vi "Run.vi"(8 "error in (no error)":errorcluster, 9 "Penalty":dbl, 10 "Maze":i32[][](array[numeric]), 11 "Runner in":refnum<class "Sentinel.lvclass">) -> (0 "error out":errorcluster, 1 "Direction":T1, 2 "Action":T2, 3 "Runner out":refnum<class "Sentinel.lvclass">, 4 "Replicated":refnum<class "Square.lvclass">)   [LabVIEW 2015, in "Sentinel.lvclass"]
uses:
  Sentinel.lvclass
  Type Defs/Action Enum.ctl
  Type Defs/Direction Enum.ctl
  Square/Square.lvclass
  Carl/Formics/Attack Options.ctl
  Sentinel.lvclass/Sentinel.ctl
  SubVIs/Read-Only Globals.vi
  Type Defs/SB Type Defs.lvlib
  Carl/Common/Common.lvlib
  Carl/Formics/Formics.lvclass
panel:
  # "NOTICE - YOU MUST NOT REMOVE THIS NOTICE. PER THE FOLLOWING LICENSE, YOU MAY REPRODUCE THIS SOFTWARE PROVIDED YOU FOLLOW THE TERMS\nOF THE LICENSE.\n\n---BEGIN BSD LICENSE (http://opensource.org/licenses/BSD-2-Clause)---\nCopyright (c) 2015, Endigit, Inc. <robert@endigit.com>\nAll rights reserved.\n\nRedistribution and use in source and binary forms, with or without modification, are permitted provided that the following conditions are met:\n\n1. Redistributions of source code must retain the above copyright notice, this list of conditions and the following disclaimer.\n\n2. Redistributions in binary form must reproduce the above copyright notice, this list of conditions and the following disclaimer in the documentation and/or other \nmaterials provided with the distribution.\n\nTHIS SOFTWARE IS PROVIDED BY THE COPYRIGHT HOLDERS AND CONTRIBUTORS \"AS IS\" AND ANY EXPRESS OR IMPLIED WARRANTIES, INCLUDING, BUT NOT \nLIMITED TO, THE IMPLIED WARRANTIES OF MERCHANTABILITY AND FITNESS FOR A PARTICULAR PURPOSE ARE DISCLAIMED. IN NO EVENT SHALL THE COPYRIGHT \nHOLDER OR CONTRIBUTORS BE LIABLE FOR ANY DIRECT, INDIRECT, INCIDENTAL, SPECIAL, EXEMPLARY, OR CONSEQUENTIAL DAMAGES (INCLUDING, BUT NOT \nLIMITED TO, PROCUREMENT OF SUBSTITUTE GOODS OR SERVICES; LOSS OF USE, DATA, OR PROFITS; OR BUSINESS INTERRUPTION) HOWEVER CAUSED AND ON \nANY THEORY OF LIABILITY, WHETHER IN CONTRACT, STRICT LIABILITY, OR TORT (INCLUDING NEGLIGENCE OR OTHERWISE) ARISING IN ANY WAY OUT OF THE USE \nOF THIS SOFTWARE, EVEN IF ADVISED OF THE POSSIBILITY OF SUCH DAMAGE.\n---END BSD LICENSE---"
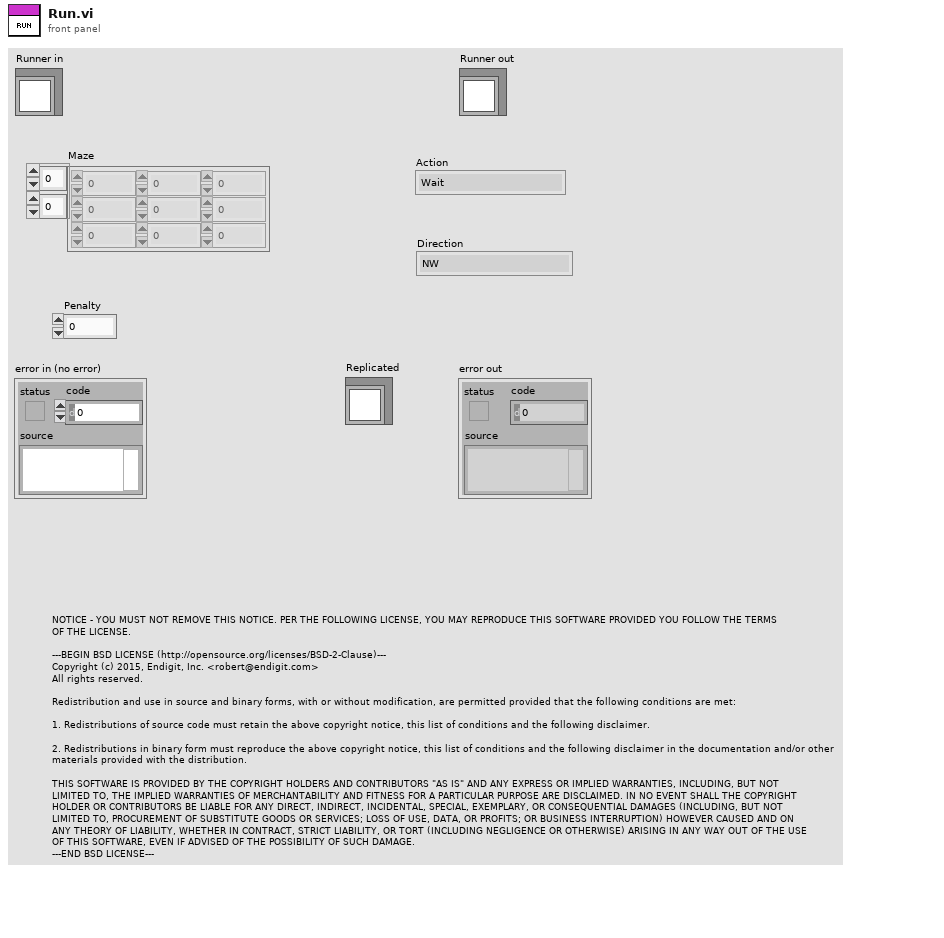
[diagram p1: front panel]
types:
  T1 = typedef "SB Type Defs.lvlib/Direction Enum.ctl" = enum16{"NW", "N", "NE", "E", "SE", "S", "SW", "W"}
  T2 = typedef "SB Type Defs.lvlib/Action Enum.ctl" = enum16{"Wait", "Move", "Attack", "Replicate"}
  T3 = typedef "Formics.lvclass/Attack Options.ctl" = enum16{"Attack", "Run", "Distract"}
  T4 = enum16{"Replicator", "Replicatee", "Eastwards", "Westwards"}
  T5 = enum16{"Replication", "Northwards", "Southwards"}
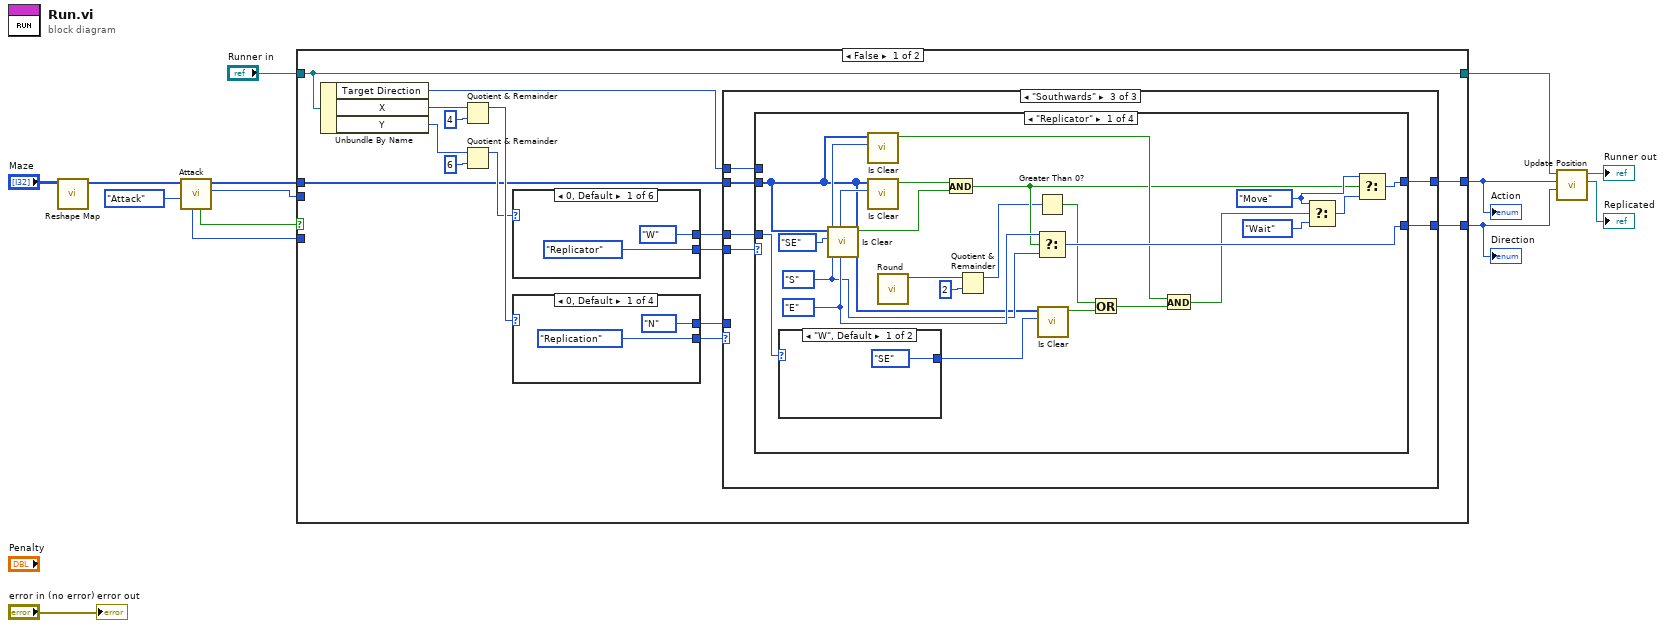
[diagram p0: block diagram]
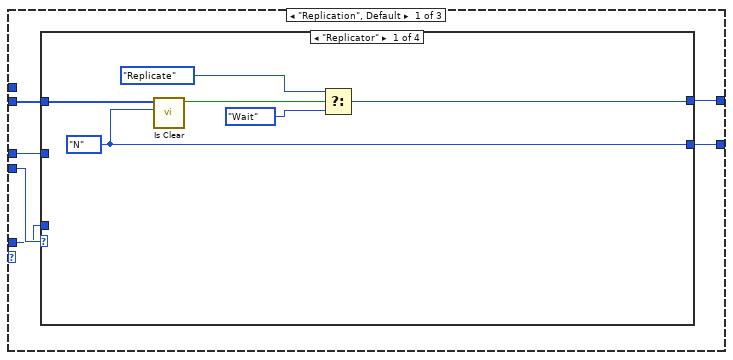
[diagram p2: hidden frame]
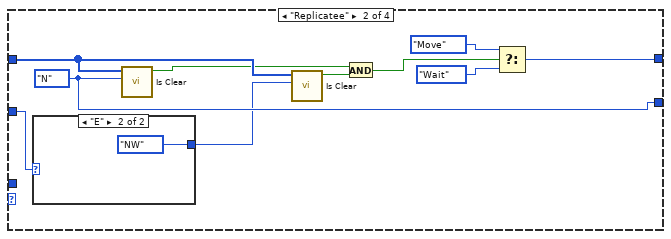
[diagram p3: hidden frame]
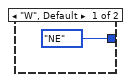
[diagram p4: hidden frame]
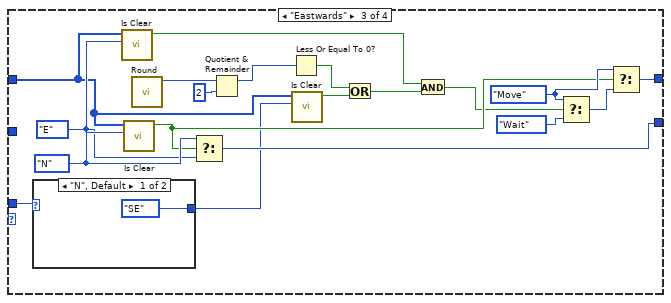
[diagram p5: hidden frame]
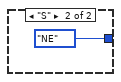
[diagram p6: hidden frame]
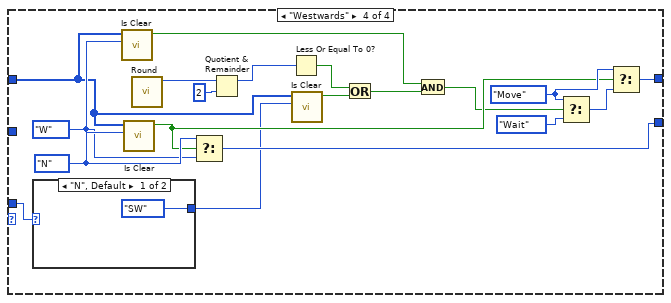
[diagram p7: hidden frame]
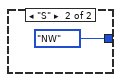
[diagram p8: hidden frame]
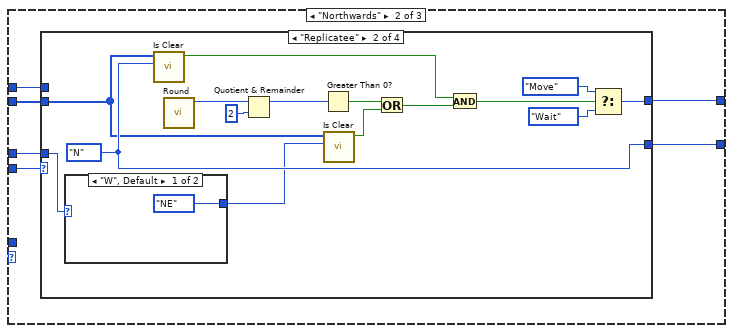
[diagram p9: hidden frame]
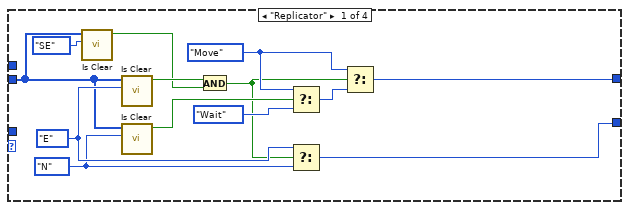
[diagram p10: hidden frame]
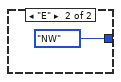
[diagram p11: hidden frame]
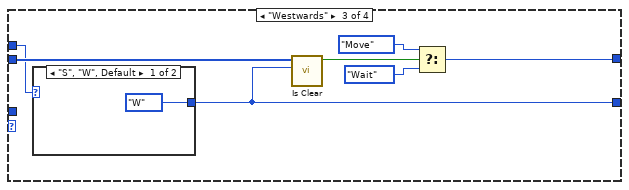
[diagram p12: hidden frame]
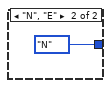
[diagram p13: hidden frame]
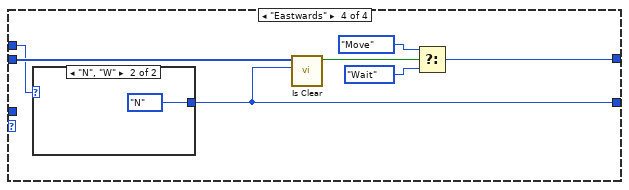
[diagram p14: hidden frame]
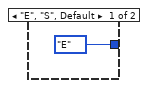
[diagram p15: hidden frame]
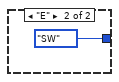
[diagram p16: hidden frame]
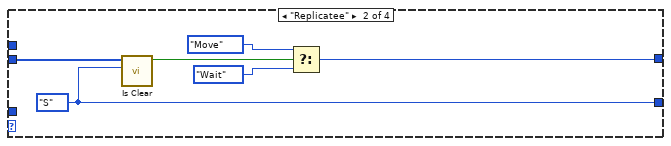
[diagram p17: hidden frame]
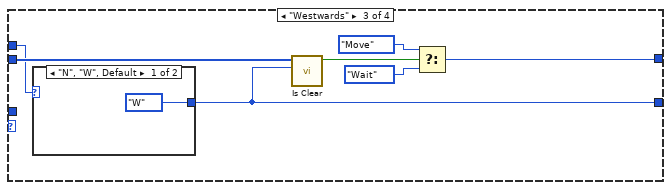
[diagram p18: hidden frame]
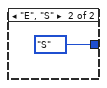
[diagram p19: hidden frame]
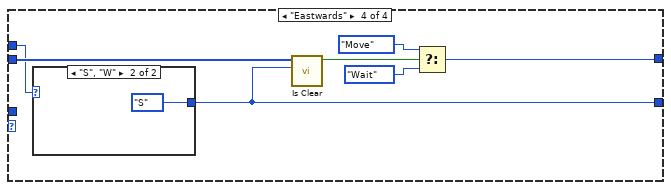
[diagram p20: hidden frame]
diagram:
  n1 = call "Reshape Map.vi"("Maze (0: Empty, -1: Enemy. >0: Teammate"="Maze") -> ("Map"=w12:i32[])  [unwired: 9 in, 1 out]
  n2 = call "Attack.vi"("Attack?"=Attack_Options."Attack", "Maze (0: Empty, -1: Enemy. >0: Teammate"=w12) -> ("Action"=w10:T2, "Maze (0: Empty, -1: Enemy. >0: Teammate 2"=w7:i32[], "Enemy Found?"=w11:bool, "Enemy Direction"=w9:i32)  [unwired: 4 in, 2 out]
  n3 = case shown="False" w11 {
    tunnel: "Runner in" -> [w21 w224]
    tunnel: w10 -> [_ w226]
    tunnel: [w20 w226] -> w1
    tunnel: w9 -> [_ w225]
    tunnel: [w19 w225] -> w2
    tunnel: [w21 w224] -> w5
    tunnel: w7 -> [w18 _]
    frame False {
      n4 = Unbundle By Name(w21) -> ("Target Direction"=w16:T1, "X"=w29:i16, "Y"=w25:i16)
      n5 = Quotient & Remainder(x=w29, y=4) -> (x-y*floor(x/y)=w27:i32)  [unwired: 1 out]
      n6 = Quotient & Remainder(x=w25, y=6) -> (x-y*floor(x/y)=w24:i32)  [unwired: 1 out]
      n7 = case shown="0, Default" w24 {
        tunnel: [T4."Replicator" ("Rows") T4."Replicatee" ("Rows") T4."Eastwards" ("Rows") T4."Replicator" ("Rows") T4."Replicatee" ("Rows") T4."Westwards" ("Rows")] -> w22
        tunnel: [Direction_Enum."W" ("Direction") Direction_Enum."E" ("Direction") Direction_Enum."E" ("Direction") Direction_Enum."E" ("Direction") Direction_Enum."W" ("Direction") Direction_Enum."W" ("Direction")] -> w17
        frame 0, Default {
        }
        frame 1 {
        }
        frame 2 {
        }
        frame 3 {
        }
        frame 4 {
        }
        frame 5 {
        }
      }
      n8 = case shown="0, Default" w27 {
        tunnel: [Direction_Enum."N" ("Direction") Direction_Enum."N" ("Direction") Direction_Enum."S" ("Direction") Direction_Enum."S" ("Direction")] -> w15
        tunnel: [T5."Replication" ("Cols") T5."Northwards" ("Cols") T5."Replication" ("Cols") T5."Southwards" ("Cols")] -> w23
        frame 0, Default {
        }
        frame 1 {
        }
        frame 2 {
        }
        frame 3 {
        }
      }
      n9 = case shown="\"Southwards\"" w23 {
        tunnel: w22 -> [w35 w101 w155]
        tunnel: [w34 w100 w154] -> w20
        tunnel: [w33 w99 w153] -> w19
        tunnel: w18 -> [w32 w98 w152]
        tunnel: w17 -> [w31 w97 w151]
        tunnel: w16 -> [_ w96 w150]
        tunnel: w15 -> [w30 _ _]
        frame "Replication", Default {
          n10 = case shown="\"Replicator\"" w35 {
            tunnel: [w38 w48 w72 w93] -> w34
            tunnel: [w40 w51 w69 w90] -> w33
            tunnel: w32 -> [w41 w46 w55 w80]
            tunnel: w31 -> [_ w47 _ _]
            tunnel: w30 -> [_ _ w54 w75]
            frame "Replicator" {
              w40 = Direction_Enum."N" ("Direction")
              n11 = call "Is Clear.vi"("Direction"=w40, "Maze (0: Empty, -1: Enemy. >0: Teammate in"=w41) -> ("Is Clear"=w36:bool)  [unwired: 9 in]
              n12 = Select(t=Action_Enum."Replicate" ("Action"), s=w36, f=Action_Enum."Wait" ("Action")) -> (s? t:f=w38:T2)
            }
            frame "Replicatee" {
              w51 = Direction_Enum."N" ("Direction")
              n13 = case shown="\"E\"" w47 {
                tunnel: [Direction_Enum."NE" ("Direction") Direction_Enum."NW" ("Direction")] -> w45
                frame "W", Default {
                }
                frame "E" {
                }
              }
              n14 = call "Is Clear.vi"("Direction"=w51, "Maze (0: Empty, -1: Enemy. >0: Teammate in"=w46) -> ("Is Clear"=w43:bool)  [unwired: 9 in]
              n15 = call "Is Clear.vi"("Direction"=w45, "Maze (0: Empty, -1: Enemy. >0: Teammate in"=w46) -> ("Is Clear"=w44:bool)  [unwired: 9 in]
              n16 = And(x=w43, y=w44) -> (x .and. y?=w42:bool)
              n17 = Select(t=Action_Enum."Move" ("Action"), s=w42, f=Action_Enum."Wait" ("Action")) -> (s? t:f=w48:T2)
            }
            frame "Eastwards" {
              w70 = Direction_Enum."E" ("Direction")
              w67 = Action_Enum."Move" ("Action")
              w71 = Direction_Enum."N" ("Direction")
              n18 = case shown="\"N\", Default" w54 {
                tunnel: [Direction_Enum."SE" ("Direction") Direction_Enum."NE" ("Direction")] -> w60
                frame "N", Default {
                }
                frame "S" {
                }
              }
              n19 = call "Is Clear.vi"("Direction"=w70, "Maze (0: Empty, -1: Enemy. >0: Teammate in"=w55) -> ("Is Clear"=w59:bool)  [unwired: 9 in]
              n20 = call "Is Clear.vi"("Direction"=w71, "Maze (0: Empty, -1: Enemy. >0: Teammate in"=w55) -> ("Is Clear"=w65:bool)  [unwired: 9 in]
              n21 = call "Round.vi"() -> ("Round"=w64:i32)  [unwired: 11 in]
              n22 = Select(t=w71, s=w65, f=w70) -> (s? t:f=w69:T1)
              n23 = Quotient & Remainder(x=w64, y=2) -> (x-y*floor(x/y)=w62:i32)  [unwired: 1 out]
              n24 = Less Or Equal To 0?(x=w62) -> (x <= 0?=w61:bool)
              n25 = call "Is Clear.vi"("Direction"=w60, "Maze (0: Empty, -1: Enemy. >0: Teammate in"=w55) -> ("Is Clear"=w58:bool)  [unwired: 9 in]
              n26 = Or(x=w61, y=w58) -> (x .or. y?=w57:bool)
              n27 = And(x=w59, y=w57) -> (x .and. y?=w56:bool)
              n28 = Select(t=w67, s=w56, f=Action_Enum."Wait" ("Action")) -> (s? t:f=w66:T2)
              n29 = Select(t=w67, s=w65, f=w66) -> (s? t:f=w72:T2)
            }
            frame "Westwards" {
              w91 = Direction_Enum."W" ("Direction")
              w88 = Action_Enum."Move" ("Action")
              w92 = Direction_Enum."N" ("Direction")
              n30 = case shown="\"N\", Default" w75 {
                tunnel: [Direction_Enum."SW" ("Direction") Direction_Enum."NW" ("Direction")] -> w81
                frame "N", Default {
                }
                frame "S" {
                }
              }
              n31 = call "Is Clear.vi"("Direction"=w91, "Maze (0: Empty, -1: Enemy. >0: Teammate in"=w80) -> ("Is Clear"=w79:bool)  [unwired: 9 in]
              n32 = call "Is Clear.vi"("Direction"=w92, "Maze (0: Empty, -1: Enemy. >0: Teammate in"=w80) -> ("Is Clear"=w86:bool)  [unwired: 9 in]
              n33 = call "Round.vi"() -> ("Round"=w84:i32)  [unwired: 11 in]
              n34 = Select(t=w92, s=w86, f=w91) -> (s? t:f=w90:T1)
              n35 = Quotient & Remainder(x=w84, y=2) -> (x-y*floor(x/y)=w83:i32)  [unwired: 1 out]
              n36 = Less Or Equal To 0?(x=w83) -> (x <= 0?=w82:bool)
              n37 = call "Is Clear.vi"("Direction"=w81, "Maze (0: Empty, -1: Enemy. >0: Teammate in"=w80) -> ("Is Clear"=w78:bool)  [unwired: 9 in]
              n38 = Or(x=w82, y=w78) -> (x .or. y?=w77:bool)
              n39 = And(x=w79, y=w77) -> (x .and. y?=w76:bool)
              n40 = Select(t=w88, s=w76, f=Action_Enum."Wait" ("Action")) -> (s? t:f=w87:T2)
              n41 = Select(t=w88, s=w86, f=w87) -> (s? t:f=w93:T2)
            }
          }
        }
        frame "Northwards" {
          n42 = case shown="\"Replicatee\"" w101 {
            tunnel: [w109 w126 w135 w144] -> w100
            tunnel: [w110 w127 w132 w141] -> w99
            tunnel: w98 -> [w108 w125 w134 w143]
            tunnel: w97 -> [_ w123 _ _]
            tunnel: w96 -> [_ _ w133 w142]
            frame "Replicator" {
              w103 = Direction_Enum."N" ("Direction")
              w111 = Direction_Enum."E" ("Direction")
              w106 = Action_Enum."Move" ("Action")
              n43 = call "Is Clear.vi"("Direction"=Direction_Enum."SE", "Maze (0: Empty, -1: Enemy. >0: Teammate in"=w108) -> ("Is Clear"=w112:bool)  [unwired: 9 in]
              n44 = call "Is Clear.vi"("Direction"=w111, "Maze (0: Empty, -1: Enemy. >0: Teammate in"=w108) -> ("Is Clear"=w113:bool)  [unwired: 9 in]
              n45 = call "Is Clear.vi"("Direction"=w103, "Maze (0: Empty, -1: Enemy. >0: Teammate in"=w108) -> ("Is Clear"=w105:bool)  [unwired: 9 in]
              n46 = And(x=w113, y=w112) -> (x .and. y?=w102:bool)
              n47 = Select(t=w106, s=w105, f=Action_Enum."Wait" ("Action")) -> (s? t:f=w104:T2)
              n48 = Select(t=w111, s=w102, f=w103) -> (s? t:f=w110:T1)
              n49 = Select(t=w106, s=w102, f=w104) -> (s? t:f=w109:T2)
            }
            frame "Replicatee" {
              w127 = Direction_Enum."N" ("Direction")
              n50 = case shown="\"W\", Default" w123 {
                tunnel: [Direction_Enum."NE" ("Direction") Direction_Enum."NW" ("Direction")] -> w122
                frame "W", Default {
                }
                frame "E" {
                }
              }
              n51 = call "Is Clear.vi"("Direction"=w127, "Maze (0: Empty, -1: Enemy. >0: Teammate in"=w125) -> ("Is Clear"=w124:bool)  [unwired: 9 in]
              n52 = call "Round.vi"() -> ("Round"=w120:i32)  [unwired: 11 in]
              n53 = Quotient & Remainder(x=w120, y=2) -> (x-y*floor(x/y)=w117:i32)  [unwired: 1 out]
              n54 = Greater Than 0?(x=w117) -> (x > 0?=w116:bool)
              n55 = call "Is Clear.vi"("Direction"=w122, "Maze (0: Empty, -1: Enemy. >0: Teammate in"=w125) -> ("Is Clear"=w118:bool)  [unwired: 9 in]
              n56 = Or(x=w116, y=w118) -> (x .or. y?=w115:bool)
              n57 = And(x=w124, y=w115) -> (x .and. y?=w121:bool)
              n58 = Select(t=Action_Enum."Move" ("Action"), s=w121, f=Action_Enum."Wait" ("Action")) -> (s? t:f=w126:T2)
            }
            frame "Westwards" {
              n59 = case shown="\"S\", \"W\", Default" w133 {
                tunnel: [Direction_Enum."W" ("Direction") Direction_Enum."N" ("Direction")] -> w132
                frame "S", "W", Default {
                }
                frame "N", "E" {
                }
              }
              n60 = call "Is Clear.vi"("Direction"=w132, "Maze (0: Empty, -1: Enemy. >0: Teammate in"=w134) -> ("Is Clear"=w136:bool)  [unwired: 9 in]
              n61 = Select(t=Action_Enum."Move" ("Action"), s=w136, f=Action_Enum."Wait" ("Action")) -> (s? t:f=w135:T2)
            }
            frame "Eastwards" {
              n62 = case shown="\"N\", \"W\"" w142 {
                tunnel: [Direction_Enum."E" ("Direction") Direction_Enum."N" ("Direction")] -> w141
                frame "E", "S", Default {
                }
                frame "N", "W" {
                }
              }
              n63 = call "Is Clear.vi"("Direction"=w141, "Maze (0: Empty, -1: Enemy. >0: Teammate in"=w143) -> ("Is Clear"=w145:bool)  [unwired: 9 in]
              n64 = Select(t=Action_Enum."Move" ("Action"), s=w145, f=Action_Enum."Wait" ("Action")) -> (s? t:f=w144:T2)
            }
          }
        }
        frame "Southwards" {
          n65 = case shown="\"Replicator\"" w155 {
            tunnel: [w172 w182 w189 w198] -> w154
            tunnel: [w173 w183 w186 w195] -> w153
            tunnel: w152 -> [w167 w181 w188 w197]
            tunnel: w151 -> [w164 _ _ _]
            tunnel: w150 -> [_ _ w187 w196]
            frame "Replicator" {
              w168 = Direction_Enum."S" ("Direction")
              w174 = Direction_Enum."E" ("Direction")
              w170 = Action_Enum."Move" ("Action")
              n66 = case shown="\"W\", Default" w164 {
                tunnel: [Direction_Enum."SE" ("Direction") Direction_Enum."SW" ("Direction")] -> w163
                frame "W", Default {
                }
                frame "E" {
                }
              }
              n67 = call "Is Clear.vi"("Direction"=Direction_Enum."SE", "Maze (0: Empty, -1: Enemy. >0: Teammate in"=w167) -> ("Is Clear"=w175:bool)  [unwired: 9 in]
              n68 = call "Is Clear.vi"("Direction"=w168, "Maze (0: Empty, -1: Enemy. >0: Teammate in"=w167) -> ("Is Clear"=w166:bool)  [unwired: 9 in]
              n69 = call "Is Clear.vi"("Direction"=w174, "Maze (0: Empty, -1: Enemy. >0: Teammate in"=w167) -> ("Is Clear"=w176:bool)  [unwired: 9 in]
              n70 = call "Round.vi"() -> ("Round"=w158:i32)  [unwired: 11 in]
              n71 = And(x=w176, y=w175) -> (x .and. y?=w162:bool)
              n72 = Quotient & Remainder(x=w158, y=2) -> (x-y*floor(x/y)=w160:i32)  [unwired: 1 out]
              n73 = Greater Than 0?(x=w160) -> (x > 0?=w161:bool)
              n74 = Select(t=w174, s=w162, f=w168) -> (s? t:f=w173:T1)
              n75 = call "Is Clear.vi"("Direction"=w163, "Maze (0: Empty, -1: Enemy. >0: Teammate in"=w167) -> ("Is Clear"=w157:bool)  [unwired: 9 in]
              n76 = Or(x=w161, y=w157) -> (x .or. y?=w156:bool)
              n77 = And(x=w166, y=w156) -> (x .and. y?=w165:bool)
              n78 = Select(t=w170, s=w165, f=Action_Enum."Wait" ("Action")) -> (s? t:f=w169:T2)
              n79 = Select(t=w170, s=w162, f=w169) -> (s? t:f=w172:T2)
            }
            frame "Replicatee" {
              w183 = Direction_Enum."S" ("Direction")
              n80 = call "Is Clear.vi"("Direction"=w183, "Maze (0: Empty, -1: Enemy. >0: Teammate in"=w181) -> ("Is Clear"=w180:bool)  [unwired: 9 in]
              n81 = Select(t=Action_Enum."Move" ("Action"), s=w180, f=Action_Enum."Wait" ("Action")) -> (s? t:f=w182:T2)
            }
            frame "Westwards" {
              n82 = case shown="\"N\", \"W\", Default" w187 {
                tunnel: [Direction_Enum."W" ("Direction") Direction_Enum."S" ("Direction")] -> w186
                frame "N", "W", Default {
                }
                frame "E", "S" {
                }
              }
              n83 = call "Is Clear.vi"("Direction"=w186, "Maze (0: Empty, -1: Enemy. >0: Teammate in"=w188) -> ("Is Clear"=w190:bool)  [unwired: 9 in]
              n84 = Select(t=Action_Enum."Move" ("Action"), s=w190, f=Action_Enum."Wait" ("Action")) -> (s? t:f=w189:T2)
            }
            frame "Eastwards" {
              n85 = case shown="\"S\", \"W\"" w196 {
                tunnel: [Direction_Enum."E" ("Direction") Direction_Enum."S" ("Direction")] -> w195
                frame "N", "E", Default {
                }
                frame "S", "W" {
                }
              }
              n86 = call "Is Clear.vi"("Direction"=w195, "Maze (0: Empty, -1: Enemy. >0: Teammate in"=w197) -> ("Is Clear"=w199:bool)  [unwired: 9 in]
              n87 = Select(t=Action_Enum."Move" ("Action"), s=w199, f=Action_Enum."Wait" ("Action")) -> (s? t:f=w198:T2)
            }
          }
        }
      }
    }
    frame True {
    }
  }
  "Action" <- w1
  "Direction" <- w2
  n88 = call-dynamic "Update Position.vi"("Direction"=w2, "Action"=w1, "Sentinel in"=w5) -> ("Sentinel in 2"=→"Replicated":refnum<class "Sentinel.lvclass">, "Sentinel out"=→"Runner out":refnum<class "Sentinel.lvclass">)  [unwired: 6 in, 1 out]
  "error out" <- "error in (no error)"
